vi "Compute Offset Angle.vi"(9 "Field of view":dbl=47.0 format="%#_13g", 11 "Offset Normilized":dbl format="%#_13g") -> (3 "Offset Angle":dbl=569.258018632146)   [LabVIEW 2025]
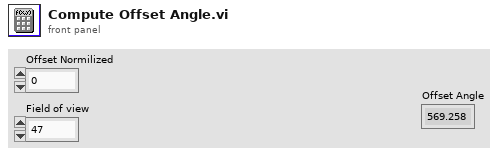
[diagram p1: front panel]
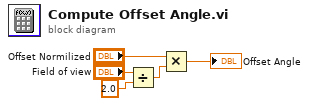
[diagram p0: block diagram]
diagram:
  n1 = Divide(x="Field of view", y=2.0) -> (x/y=w2:dbl)
  n2 = Multiply(x="Offset Normilized", y=w2) -> (x*y=→"Offset Angle":dbl)
